vi "UID to Reference.vi"(10 "Error In":errorcluster, 11 "UID":i32) -> (2 "Error Out":errorcluster, 3 "GObj Refnum":refnum<vi>)   [LabVIEW 2019]
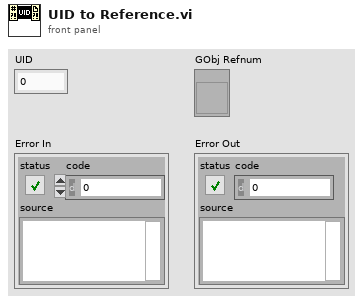
[diagram p1: front panel]
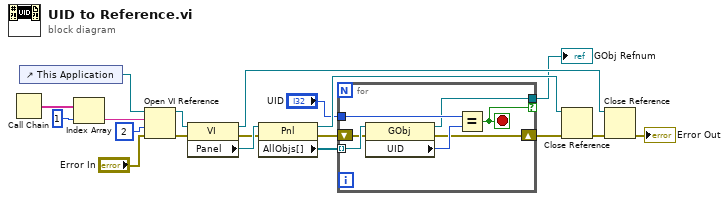
[diagram p0: block diagram]
diagram:
  n1 = Call Chain() -> (call chain=w16:string[])
  n2 = control-ref of="This Application"() -> (w1:refnum<vi>)
  n3 = Index Array(array=w16, index=1 ("Index")) -> (element=w18:string)
  n4 = Open VI Reference(application reference (local)=w1, vi path=w18, options=2, error in (no error)="Error In") -> (vi reference=w15:refnum<vi>, error out=w8:errorcluster)  [unwired: 2 in]
  n5 = property class="VI"(reference=w15, error in=w8) -> (reference out=w13:refnum<vi>, error out=w7:errorcluster, "Panel"=w14:refnum<vi>)
  n6 = property class="Pnl"(reference=w14, error in=w7) -> (reference out=w12:refnum<vi>, error out=w6:errorcluster, "AllObjs[]"=w10:refnum<vi>[])
  n7 = for {
    tunnel: w10 -> [w26] mode=indexing
    tunnel: "UID" -> [w25]
    tunnel: [w23] -> w4 if=w22
    shift-right: [w20] -> w5
    shift-left: w6 -> [w21]
    stop <- w22 stop-if-true
    n8 = property class="GObj"(reference=w26, error in=w21) -> (reference out=w23:refnum<vi>, error out=w20:errorcluster, "UID"=w24:i32)
    n9 = Equal?(x=w25, y=w24) -> (x = y?=w22:bool)
  }
  "GObj Refnum" <- w4
  n10 = Close Reference(reference=w12, error in (no error)=w5) -> (error out=w11:errorcluster)
  n11 = Close Reference(reference=w13, error in (no error)=w11) -> (error out=→"Error Out":errorcluster)
